vi "checkFolder.vi"(0 "reference in":refnum<class "excelFile.lvclass">, 5 "error in (no error)":errorcluster) -> (14 "reference out":refnum<class "excelFile.lvclass">, 16 "backup_path":path, 19 "error out":errorcluster)   [LabVIEW 2016, in "excelFile.lvclass"]
uses:
  excelFile.lvclass
  <vilib>/Utility/sysdir.llb/System Directory Type.ctl
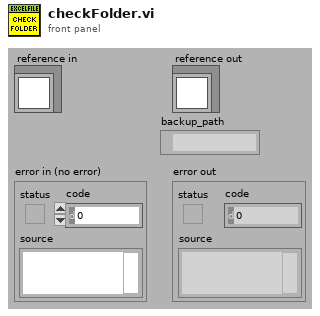
[diagram p1: front panel]
types:
  T1 = typedef "System Directory Type.ctl" = i32
  T2 = typedef "excelFile.lvclass/ObjectAttributesRef.ctl" = refnum<data-value>
  T3 = typedef "excelFile.lvclass/ObjectAttributes.ctl" = cluster{"MyAttribute":dbl, "path":string, "Refnum Excel":cluster{"Excel._Application":refnum<k7>, "Workbooks":refnum<k7>, "Open":refnum<k7>}, "data":string[][][], "save":bool, "fileType":T4, "rowsColor":u32[], "python_ref":refnum<class "python.lvclass">, "items_rows":i32[], "excel_range":i32[][], "TSR":cluster{"number":string, "TSR_path":path, "service_path":path, "email_to":string}, "excel_already_opened?":bool, "file_already_opened?":bool, "excel_protected_opened?":bool, "Refnum Cluster Worksheets":cluster{"Excel._Application":refnum<k7>, "Workbooks":refnum<k7>, "Open":refnum<k7>, "Worksheets":refnum<k7>, "Excel._Worksheet":refnum<k7>}, "#_rows_defective":i32, "#_rows_spare":i32}
  T4 = typedef "excelFile.lvclass/fileType.ctl" = enum16{"devices", "items", "partsTracking", "TSR"}
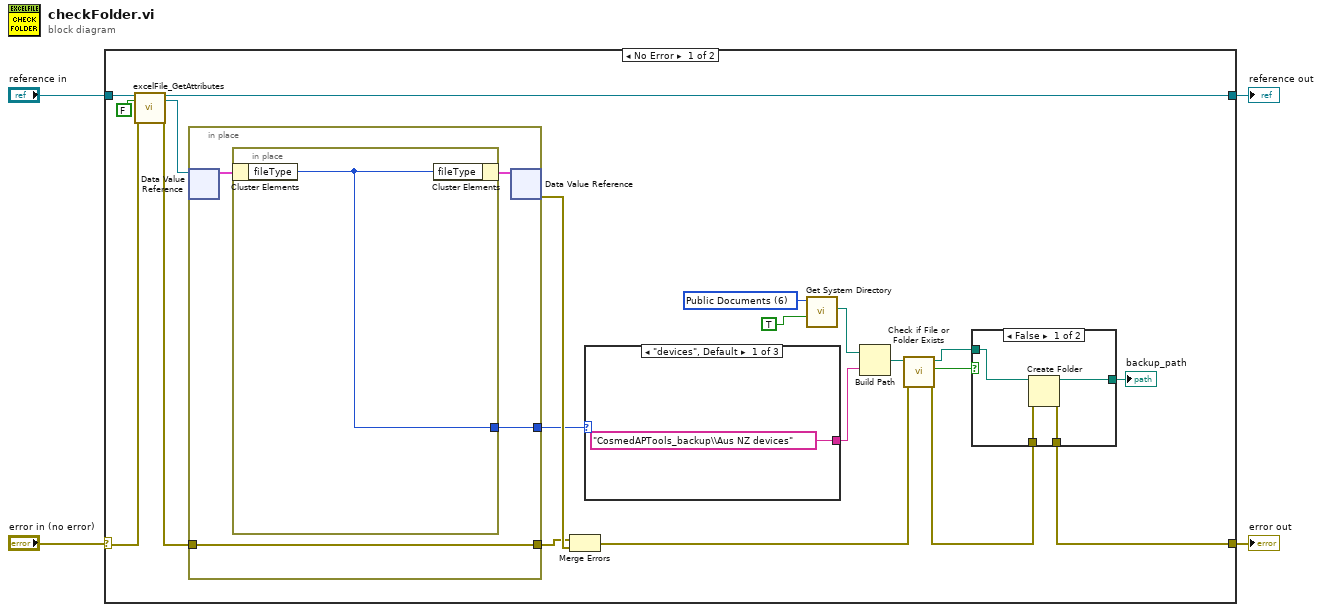
[diagram p0: block diagram]
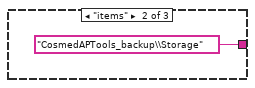
[diagram p3: hidden frame]
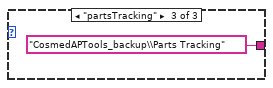
[diagram p4: hidden frame]
diagram:
  n1 = case shown="No Error" "error in (no error)" {
    selector: "error in (no error)" -> [w20 w40]
    tunnel: [w7 w40] -> w3
    tunnel: [w18 w39] -> w1
    tunnel: "reference in" -> [w22 w39]
    frame No Error {
      w16 = T1 6 items=["User Home"=0, "User Desktop"=1, "User Documents"=2, "User Application Data"=3, "User Preferences"=4, "User Temporary"=5, "Public Documents"=6, "Public Application Data"=7, "Public Preferences"=8, "Public Cache"=13, "System Core Libraries"=9, "System Installed Libraries"=10, "Application Files"=11, "Boot Volume Root"=12] ("system directory type")
      n2 = call "excelFile_GetAttributes.vi"("reference in"=w22, "return data? (T)"=FALSE, "error in (no error)"=w20) -> ("reference out"=w18:refnum<class "excelFile.lvclass">, "attributes ref"=w17:T2, "error out"=w19:errorcluster)  [unwired: 13 in, 1 out]
      n3 = in-place {
        in-place-border: w19 -> [w35]
        in-place-border: [w35] -> w23
        in-place-border: [w34] -> w13
        n4 = in-place-dvr #1(w17) -> (w36:T3)  [unwired: 1 out]
        n5 = in-place {
          in-place-border: [w38] -> w34
          n6 = in-place-cluster #2(w36) -> ("fileType"=w38:T4)
          n7 = in-place-cluster #2("fileType"=w38) -> (w37:T3)
        }
        n8 = in-place-dvr #1(w37) -> (w24:errorcluster)  [unwired: 1 out]
      }
      n9 = Merge Errors(w23, w24) -> (w9:errorcluster)
      n10 = case shown="\"devices\", Default" w13 {
        tunnel: ["CosmedAPTools_backup\\Aus NZ devices" ("name or relative path") "CosmedAPTools_backup\\Storage" ("name or relative path") "CosmedAPTools_backup\\Parts Tracking" ("name or relative path")] -> w12
        frame "devices", Default {
        }
        frame "items" {
        }
        frame "partsTracking" {
        }
      }
      n11 = call <vilib>:"Get System Directory.vi"("create directory if not found? (F)"=TRUE, "system directory type"=w16) -> ("system directory"=w14:path)  [unwired: 9 in]
      n12 = Build Path(base path=w14, name or relative path=w12) -> (appended path=w11:path)
      n13 = call <vilib>:"Check if File or Folder Exists.vi"("error in (no error)"=w9, "path"=w11) -> ("error out"=w8:errorcluster, "file or folder exists?"=w10:bool, "dup path"=w6:path)  [unwired: 7 in]
      n14 = case shown="False" w10 {
        tunnel: w8 -> [w28 w29]
        tunnel: [w27 w29] -> w7
        tunnel: w6 -> [w26 w30]
        tunnel: [w25 w30] -> w5
        frame False {
          n15 = Create Folder(path (use dialog)=w26, error in=w28) -> (created path=w25:path, error out=w27:errorcluster)  [unwired: 1 in, 1 out]
        }
        frame True {
        }
      }
      "backup_path" <- w5
    }
    frame Error {
    }
  }
  "error out" <- w3
  "reference out" <- w1
